vi "Taller1_LecturaSonido.vi"() -> ()   [LabVIEW 2022 SP3]
uses:
  <vilib>/express/express analysis/Spectral/Block/exnSpectralBlock spectral measurements peak poly.vi
  <vilib>/express/express analysis/Spectral/Block/exnSpectralBlock spectral measurements peak WFM.vi
  <vilib>/express/express analysis/Spectral/XNode/ExpressSpectralMeasurementsBlockNode.xnode
  <vilib>/Analysis/2dsp.llb/Real FFT.vi
  <vilib>/Analysis/NI_AALPro.lvlib
panel:
  out "Espectro":cluster{"f0":dbl, "df":dbl, "magnitude":dbl[]}(graph)
  out "FFT":dbl[](graph)
  out "Audio Signal":waveform(dbl)[](graph)
  out "Samples":i32
  in  "number of samples/ch (-1: all)":i32=-1
  in  "path":path
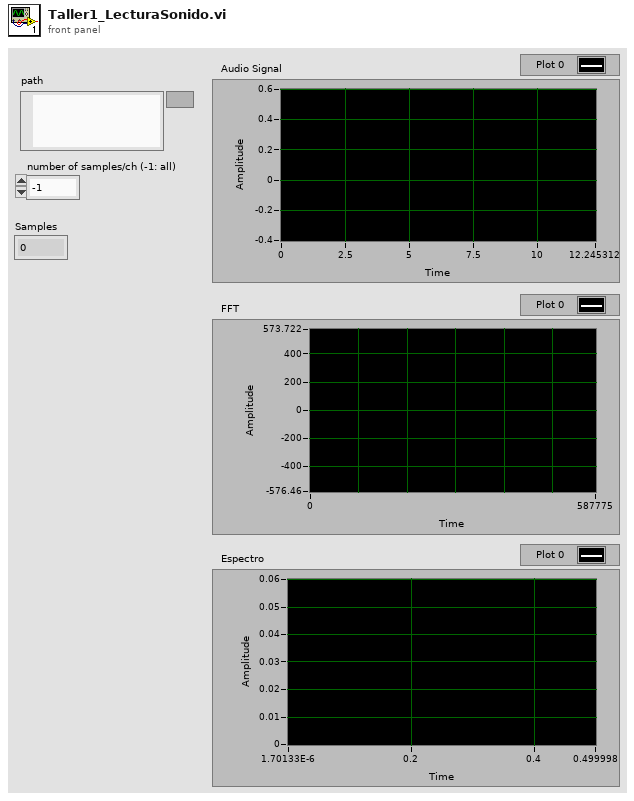
[diagram p1: front panel]
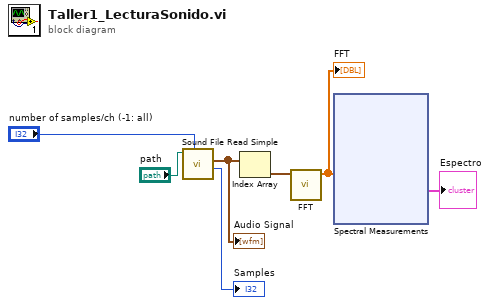
[diagram p0: block diagram]
diagram:
  n1 = call <vilib>:"Sound File Read Simple.vi"("number of samples/ch (-1: all)"="number of samples/ch (-1: all)", "path"="path") -> ("offset"=→"Samples":i32, "data"=w3:waveform(dbl)[])  [unwired: 6 in, 2 out]
  "Audio Signal" <- w3
  n2 = Index Array(array=w3) -> (element=w4:waveform(dbl))  [unwired: 1 in]
  n3 = call-poly <vilib>:"FFT.vi"("X"=w4) -> ("FFT {X}"=w2:cdb[])  [unwired: 9 in, 1 out]
  "FFT" <- w2
  n4 = xnode "Spectral Measurements"("Signals"=w2) -> ("FFT - (Peak)"=→"Espectro":cluster{"f0":dbl, "df":dbl, "magnitude":dbl[]})  [unwired: 1 in, 2 out]
